vi "NextStateCheck.vi"(8 "Error In":errorcluster, 10 "Current State":T1, 11 "Queue":refnum<queue>) -> (0 "Error Out":errorcluster, 3 "Checked State":T1)   [LabVIEW 2010]
uses:
  States.ctl
panel:
  # "Outputs"
  # "Inputs"
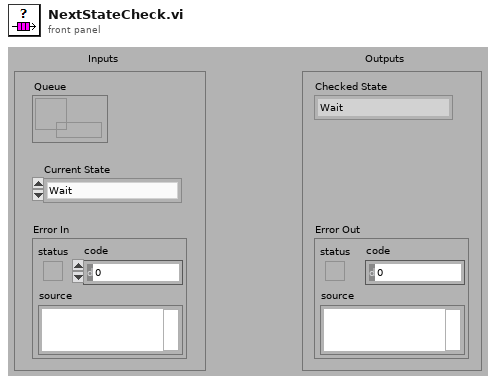
[diagram p1: front panel]
types:
  T1 = typedef "States.ctl" = enum16{"Wait", "Initialize", "Read Port", "Write Port", "Close"}
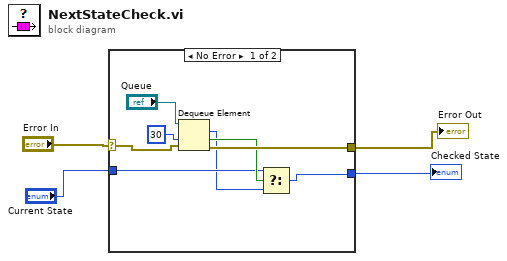
[diagram p0: block diagram]
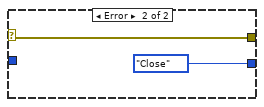
[diagram p2: hidden frame]
diagram:
  n1 = case shown="No Error" "Error In" {
    selector: "Error In" -> [w11 w13]
    tunnel: [w10 w13] -> w3
    tunnel: [w6 States."Close" ("Enum")] -> w2
    tunnel: "Current State" -> [w8 _]
    frame No Error {
      n2 = Dequeue Element(queue="Queue", timeout in ms (-1)=30, error in (no error)=w11) -> (element=w7:T1, timed out?=w9:bool, error out=w10:errorcluster)  [unwired: 1 out]
      n3 = Select(t=w8, s=w9, f=w7) -> (s? t:f=w6:T1)
    }
    frame Error {
    }
  }
  "Checked State" <- w2
  "Error Out" <- w3
